vi "Main_UI.vi"   [LabVIEW 2019]
uses:
  Global Plantita Parameters.vi
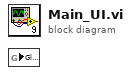
[diagram p0: block diagram]
diagram:
  n1 = global read "Global Plantita Parameters.vi" item#-1() -> ()  [unwired: 1 in]
